vi "Front Panel Show.vi"(8 "error in":errorcluster, 11 "last level":i32=1) -> (0 "error out":errorcluster)   [LabVIEW 2020]
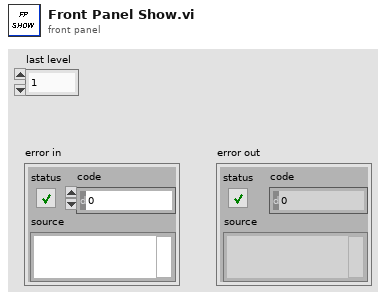
[diagram p1: front panel]
types:
  T1 = enum32{"Invalid", "Standard", "Closed", "Hidden", "Minimized", "Maximized"}
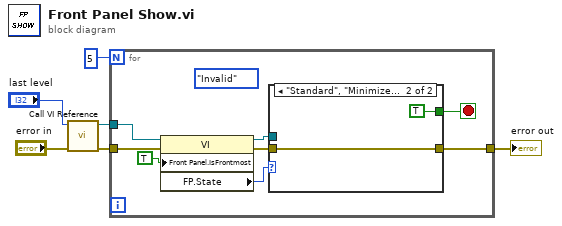
[diagram p0: block diagram]
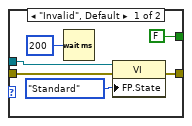
[diagram p2: hidden frame]
diagram:
  n1 = call "Call VI Reference.vi"("error in"="error in", "last level"="last level") -> ("error out"=w1:errorcluster, "vi reference out"=w5:refnum<vi>)  [unwired: 8 in]
  n2 = for {
    N: 5 -> [_]
    tunnel: w5 -> [w13]
    tunnel: w1 -> [w9]
    tunnel: [w7] -> w3
    stop <- w10 stop-if-true
    (unwired) T1."Invalid" ("Front Panel Window:State")
    n3 = property class="VI"(reference=w13, error in=w9, "Front Panel.IsFrontmost"=TRUE ("Front Panel Window:Is Frontmost")) -> (reference out=w11:refnum<vi>, error out=w8:errorcluster, "FP.State"=w12:T1)
    n4 = case shown="\"Standard\", \"Minimized\", \"Maximized\"" w12 {
      tunnel: w11 -> [w20 _]
      tunnel: [FALSE TRUE] -> w10
      tunnel: w8 -> [w16 w21]
      tunnel: [w15 w21] -> w7
      frame "Invalid", Default {
        n5 = Wait (ms)(milliseconds to wait=u32 200) -> ()  [unwired: 1 out]
        n6 = property class="VI"(reference=w20, error in=w16, "FP.State"=T1."Standard" ("Front Panel Window:State")) -> (error out=w15:errorcluster)  [unwired: 1 out]
      }
      frame "Standard", "Minimized", "Maximized" {
      }
    }
  }
  "error out" <- w3
